vi "Linker.Remove sub tests.vi"(10 "Linker.Read Info From File":T2(array[cluster]), 11 "Tests":path[](array[path])) -> (3 "Array":path[](array[path]))   [LabVIEW 2013, in "Caraya.lvlib" / "Test Runner.lvclass"]
uses:
  Test Runner/Test Runner.lvclass
  <vilib>/Utility/lvfile.llb/LVFileType.ctl
  <vilib>/Utility/lvfile.llb/NI_FileType.lvlib
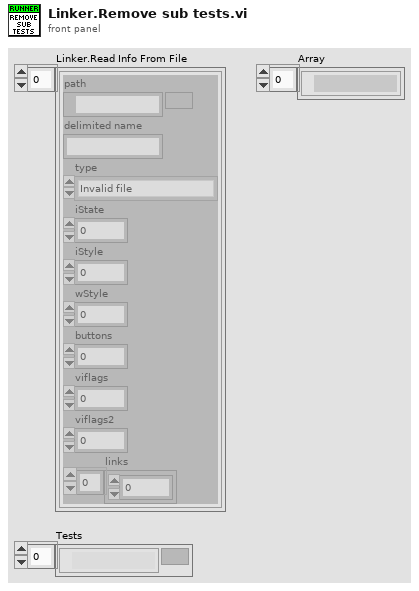
[diagram p1: front panel]
types:
  T1 = typedef "NI_FileType.lvlib/LVFileType.ctl" = enum32{"Invalid file", "Unknown type", "Instrument", "Control", "Polymorphic VI", "Project", "Library", "LVClass", "XControl", "XNode", "Shared library", ".NET assembly", "ActiveX interface", "CIN", "Run-time menu", "Palette menu", "Help file", "LLB", "XNode Edit Dependency", "Class Private Data Control", "Statechart", "MathScript .m file", "Ladder Diagram", "LVLibp", "XNode Build Dependency"}
  T2 = cluster{"path":path, "delimited name":string, "type":T1, "iState":u32, "iStyle":u16, "wStyle":u16, "buttons":u16, "viflags":u32, "viflags2":u32, "links":u32[]}[]
  T3 = cluster{"path":path, "delimited name":string, "type":T1, "iState":u32, "iStyle":u16, "wStyle":u16, "buttons":u16, "viflags":u32, "viflags2":u32, "links":u32[]}
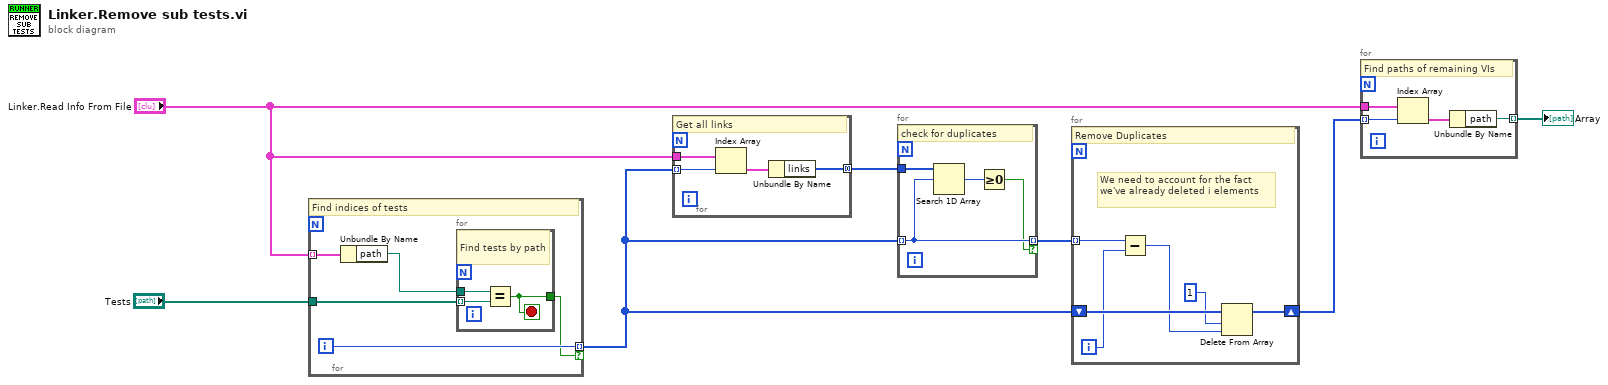
[diagram p0: block diagram]
diagram:
  n1 = for {
    tunnel: "Linker.Read Info From File" -> [w12] mode=indexing
    tunnel: "Tests" -> [w10]
    tunnel: [w9] -> w4 mode=indexing if=w8
    i -> [w9]
    # "Find indices of tests"
    n2 = Unbundle By Name(w12) -> ("path"=w11:path)
    n3 = for {
      tunnel: w11 -> [w15]
      tunnel: w10 -> [w14] mode=indexing
      tunnel: [w13] -> w8
      stop <- w13 stop-if-true
      # "Find tests by path"
      n4 = Equal?(x=w15, y=w14) -> (x = y?=w13:bool)
    }
  }
  n5 = for {
    tunnel: w4 -> [w18] mode=indexing
    tunnel: "Linker.Read Info From File" -> [w19]
    tunnel: [w16] -> w2 mode=concatenating
    # "Get all links"
    n6 = Index Array(array=w19, index=w18) -> (element=w17:T3)
    n7 = Unbundle By Name(w17) -> ("links"=w16:u32[])
  }
  n8 = for {
    tunnel: w2 -> [w23]
    tunnel: w4 -> [w21] mode=indexing
    tunnel: [w21] -> w3 mode=indexing if=w20
    # "check for duplicates"
    n9 = Search 1D Array(1D array=w23, element=w21) -> (index of element=w22:i32)  [unwired: 1 in]
    n10 = Greater Or Equal To 0?(x=w22) -> (x >= 0?=w20:bool)
  }
  n11 = for {
    tunnel: w3 -> [w28] mode=indexing
    shift-right: [w24] -> w5
    shift-left: w4 -> [w29]
    i -> [w27]
    # "We need to account for the fact we've already deleted i elements"
    # "Remove Duplicates"
    n12 = Subtract(x=w28, y=w27) -> (x-y=w26:i32)
    n13 = Delete From Array(array=w29, length=1, index=w26) -> (array with subset deleted=w24:i32[])  [unwired: 1 out]
  }
  n14 = for {
    tunnel: w5 -> [w32] mode=indexing
    tunnel: "Linker.Read Info From File" -> [w33]
    tunnel: [w30] -> w7 mode=indexing
    # "Find paths of remaining VIs"
    n15 = Index Array(array=w33, index=w32) -> (element=w31:T3)
    n16 = Unbundle By Name(w31) -> ("path"=w30:path)
  }
  "Array" <- w7
